vi "7400 CANOpen OD Index not defined--error.vi"(8 "error in":errorcluster, 11 "Argument":string) -> (0 "error out":errorcluster, 2 "Error Code":i32)   [LabVIEW 2020, in "CANopen.lvlib" / "Object Dictionary.lvclass"]
uses:
  Object Dictionary.lvclass
  Object Dictionary.lvclass/Object Dictionary.ctl
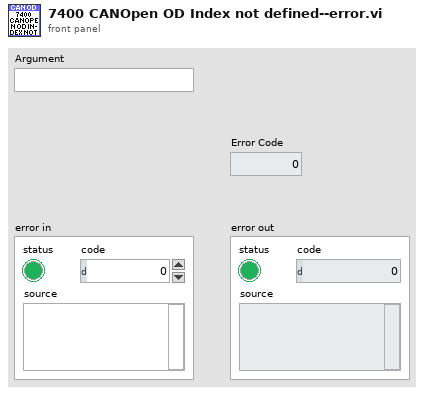
[diagram p1: front panel]
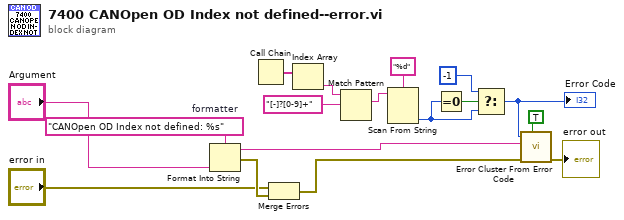
[diagram p0: block diagram]
diagram:
  w14 = "CANOpen OD Index not defined: %s"  # formatter
  n1 = Format Into String(format string=w14, "Argument") -> (resulting string=w15:string, error out=w3:errorcluster)  [unwired: 2 in]
  n2 = Call Chain() -> (call chain=w5:string[])
  n3 = Merge Errors("error in", w3) -> (w1:errorcluster)
  n4 = Index Array(array=w5) -> (element=w10:string)  [unwired: 1 in]
  n5 = Match Pattern(string=w10, regular expression="[-]?[0-9]+") -> (match substring=w11:string)  [unwired: 1 in, 3 out]
  n6 = Scan From String(format string="%d", input string=w11) -> (output 1=w7:i32)  [unwired: 3 in, 3 out]
  n7 = Equal To 0?(x=w7) -> (x = 0?=w8:bool)
  n8 = Select(t=-1, s=w8, f=w7) -> (s? t:f=w4:i32)
  "Error Code" <- w4
  n9 = call <vilib>:"Error Cluster From Error Code.vi"("show call chain? (False)"=TRUE, "error in (no error)"=w1, "error message (\"\")"=w15, "error code (0)"=w4) -> ("error out"=→"error out":errorcluster)  [unwired: 5 in]
